vi "GV_ToolbarShowTimeSpan.vi"(8 "error in (no error)":errorcluster, 11 "Gviewer in":refnum<class "Gviewer.lvclass">) -> (0 "error out":errorcluster, 1 "TimeSpanText":string, 3 "Gviewer out":refnum<class "Gviewer.lvclass">)   [LabVIEW 2020, in "Sgraph_lib_V1.lvlib" / "Gviewer.lvclass"]
doc: "Andre Koelewijn, 1 may 2021\n\nShow timespan in right side of toolbar area"
uses:
  Gviewer.lvclass
  Gviewer.lvclass/Gviewer.ctl
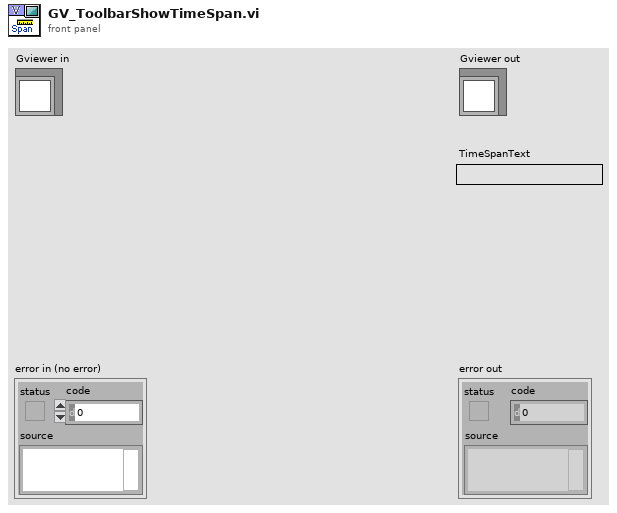
[diagram p1: front panel]
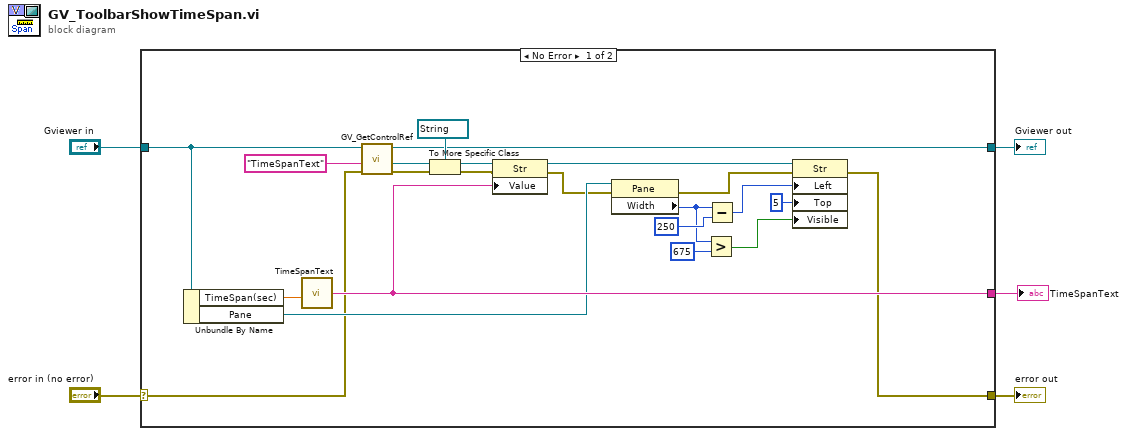
[diagram p0: block diagram]
diagram:
  n1 = case shown="No Error" "error in (no error)" {
    selector: "error in (no error)" -> [w13 w29]
    tunnel: [w12 w29] -> w4
    tunnel: [w6 w28] -> w2
    tunnel: "Gviewer in" -> [w25 w28]
    tunnel: [w24 _] -> w1
    frame No Error {
      n2 = Unbundle By Name(w25) -> ("TimeSpan(sec)"=w27:dbl, "Pane"=w18:refnum<vi>)
      n3 = call "TimeSpanText.vi"("Timespan"=w27) -> ("TimeSpanText"=w24:string)  [unwired: 4 in]
      n4 = call "GV_GetControlRef.vi"("error in (no error)"=w13, "CNT name"="TimeSpanText", "Gviewer in"=w25) -> ("error out"=w22:errorcluster, "Reference"=w23:refnum<vi>, "Gviewer out"=w6:refnum<class "Gviewer.lvclass">)  [unwired: 6 in]
      n5 = To More Specific Class(target class=refnum<vi> refnum ("TimeSpanText"), reference=w23, error in=w22) -> (specific class reference=w20:refnum<vi>, error out=w19:errorcluster)
      n6 = property class="Str"(reference=w20, error in=w19, "Value"=w24) -> (reference out=w16:refnum<vi>, error out=w17:errorcluster)
      n7 = property class="Pane"(reference=w18, error in=w17) -> (error out=w14:errorcluster, "Width"=w9:u32)  [unwired: 1 out]
      n8 = Greater?(x=w9, y=u32 675) -> (0:w7:bool)
      n9 = Subtract(x=w9, y=u32 250) -> (x-y=w11:u32)
      n10 = property class="Str"(reference=w16, error in=w14, "Left"=w11, "Top"=5 ("Position:Top"), "Visible"=w7) -> (error out=w12:errorcluster)  [unwired: 1 out]
    }
    frame Error {
    }
  }
  "error out" <- w4
  "Gviewer out" <- w2
  "TimeSpanText" <- w1
